vi "GenerateDictt.vi"(10 "Stop":dbl, 11 "Start":dbl) -> (3 "Array":dbl[][](array[numeric]))   [LabVIEW 2018]
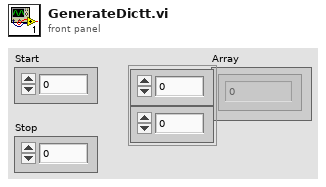
[diagram p1: front panel]
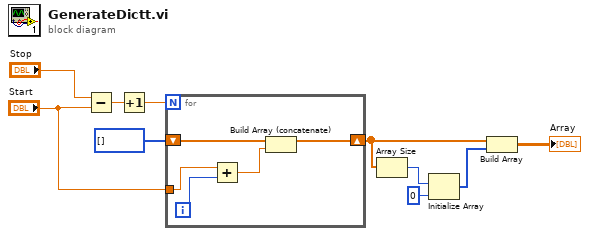
[diagram p0: block diagram]
diagram:
  n1 = Subtract(x="Stop", y="Start") -> (x-y=w2:dbl)
  n2 = Increment(x=w2) -> (x+1=w5:dbl)
  n3 = for {
    N: w5 -> [_]
    tunnel: "Start" -> [w12]
    shift-right: [w14] -> w6
    shift-left: i32[] [] -> [w15]
    i -> [w13]
    n4 = Add(x=w12, y=w13) -> (x+y=w11:dbl)
    n5 = Build Array (concatenate)(w15, w11) -> (w14:dbl[])
  }
  n6 = Array Size(array=w6) -> (size(s)=w7:i32)
  n7 = Initialize Array(w7, 0 ("dimension size")) -> (w9:i32[])
  n8 = Build Array(w6, w9) -> (→"Array":dbl[][])
